vi "Draw Flattened Blended Pixmap.vi"(6 "error in (no error)":errorcluster, 8 "image data":T1, 9 "picture":picture) -> (0 "error out":errorcluster, 3 "new picture":picture)   [LabVIEW 2020]
doc: "Draws a 32-bit RGBA pixmap into a picture using the fourth byte to determine the alpha or transparency of each pixel."
uses:
  <vilib>/picture/picture.llb/imagedata.ctl
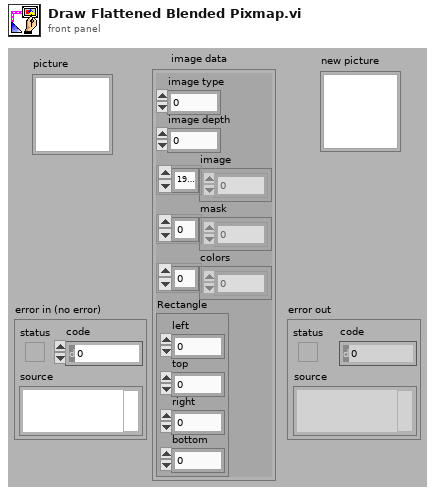
[diagram p1: front panel]
types:
  T1 = typedef "imagedata.ctl" = cluster{"image type":i32, "image depth":i32, "image":u8[], "mask":u8[], "colors":u32[], "Rectangle":cluster{"left":i16, "top":i16, "right":i16, "bottom":i16}}
  T2 = cluster{"left":i16, "top":i16, "right":i16, "bottom":i16}
  T3 = cluster{"top":i16, "left":i16, "bottom":i16, "right":i16}
  T4 = cluster{"default foreground":u32, "default background":u32}
  T5 = cluster{"opcode-Copy  Blended Pixmap":i16, i32, i32, cluster{"top":i16, "left":i16, "bottom":i16, "right":i16}, i16, cluster{"default foreground":u32, "default background":u32}}
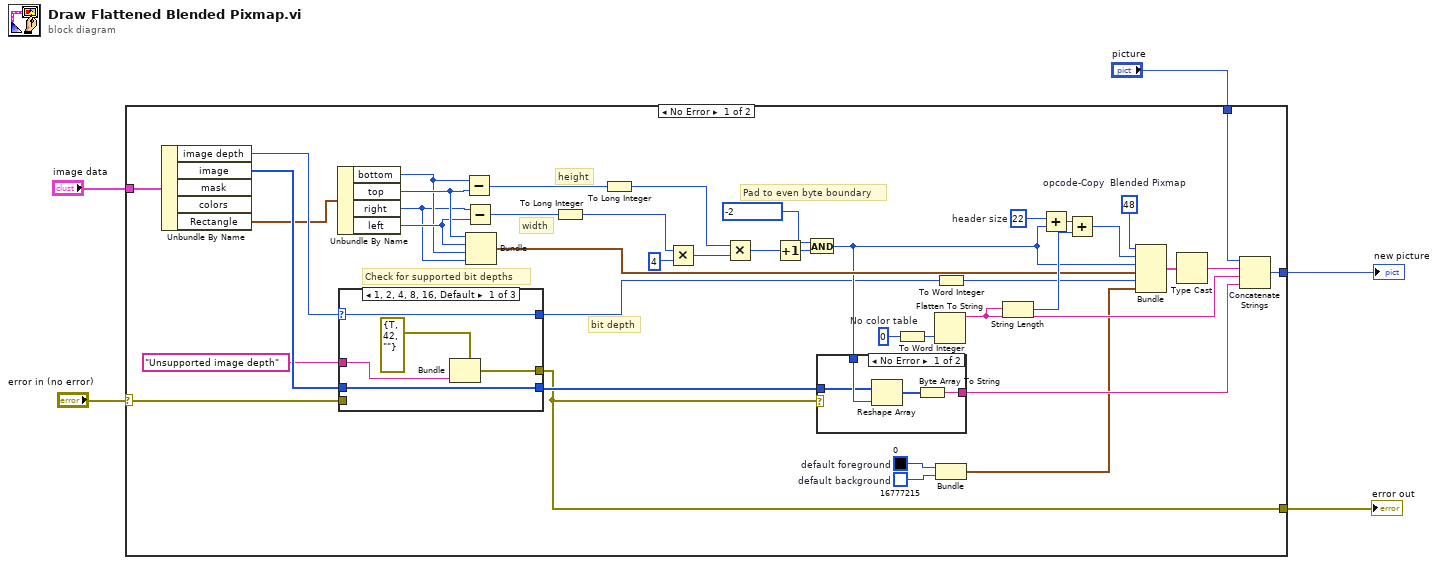
[diagram p0: block diagram]
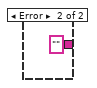
[diagram p2: hidden frame]
diagram:
  n1 = case shown="No Error" "error in (no error)" {
    selector: "error in (no error)" -> [w7 w64]
    tunnel: [w40 w63] -> w5
    tunnel: "picture" -> [w39 w63]
    tunnel: "image data" -> [w38 _]
    tunnel: [w6 w64] -> w2
    frame No Error {
      w26 = i16 22  # header size
      w24 = i16 48  # opcode-Copy  Blended Pixmap
      w31 = 0  # No color table
      w41 = u32 16777215  # default background
      w42 = u32 0  # default foreground
      # "Pad to even byte boundary"
      # "Check for supported bit depths"
      # "bit depth"
      # "height"
      # "width"
      n2 = Unbundle By Name(w38) -> ("image depth"=w36:i32, "image"=w35:u8[], "Rectangle"=w18:T2)  [unwired: 2 out]
      n3 = Unbundle By Name(w18) -> ("bottom"=w13:i16, "top"=w15:i16, "right"=w12:i16, "left"=w14:i16)
      n4 = case shown="1, 2, 4, 8, 16, Default" w36 {
        selector: w36 -> [w56 w59 w61]
        tunnel: [w56 w59 w61] -> w9
        tunnel: w35 -> [w55 w58 w62]
        tunnel: [w55 w58 w62] -> w22
        tunnel: [w52 w57 w60] -> w6
        tunnel: w7 -> [_ w57 w60]
        tunnel: "Unsupported image depth" -> [w53 _ _]
        frame 1, 2, 4, 8, 16, Default {
          n5 = Bundle(cluster=errorcluster {"status"=TRUE, "code"=42, "source"=""} ("Unsupported Image Depth error"), "source"=w53) -> (w52:errorcluster)  [unwired: 2 in]
        }
        frame 24 {
          # "Add Alpha, or let through?"
        }
        frame 32 {
        }
      }
      n6 = Subtract(x=w13, y=w15) -> (x-y=w16:i16)
      n7 = Subtract(x=w12, y=w14) -> (x-y=w17:i16)
      n8 = Bundle("top"=w15, "left"=w14, "bottom"=w13, "right"=w12) -> (w37:T3)  [unwired: 1 in]
      n9 = To Long Integer(number=w17) -> (32bit integer=w19:i32)
      n10 = To Long Integer(number=w16) -> (32bit integer=w11:i32)
      n11 = Multiply(x=w19, y=4 ("f")) -> (x*y=w21:i32)
      n12 = Multiply(x=w11, y=w21) -> (x*y=w32:i32)
      n13 = Increment(x=w32) -> (x+1=w34:i32)
      n14 = And(x=-2, y=w34) -> (x .and. y?=w23:i32)
      n15 = case shown="No Error" w6 {
        tunnel: [w50 ""] -> w44
        tunnel: w23 -> [w49 _]
        tunnel: w22 -> [w48 _]
        frame No Error {
          n16 = Reshape Array(w48, w49) -> (w47:u8[])
          n17 = Byte Array To String(unsigned byte array=w47) -> (string=w50:string)
        }
        frame Error {
        }
      }
      n18 = To Word Integer(number=w31) -> (16bit integer=w30:i16)
      n19 = Flatten To String(anything=w30) -> (data string=w45:string)  [unwired: 3 in, 2 out]
      n20 = To Word Integer(number=w9) -> (16bit integer=w10:i16)
      n21 = Bundle("default foreground"=w42, "default background"=w41) -> (w43:T4)  [unwired: 1 in]
      n22 = String Length(string=w45) -> (length=w46:i32)
      n23 = Add(x=w26, y=w23) -> (x+y=w27:i32)
      n24 = Add(x=w27, y=w46) -> (x+y=w28:i32)
      n25 = Bundle("opcode-Copy  Blended Pixmap"=w24, w28, w23, w37, w10, w43) -> (w25:T5)  [unwired: 1 in]
      n26 = Type Cast(x=w25) -> (*(type *) &x=w29:string)  [unwired: 1 in]
      n27 = Concatenate Strings(w39, w29, w45, w44) -> (w40:picture)
    }
    frame Error {
    }
  }
  "new picture" <- w5
  "error out" <- w2
